vi "Arm Controller.vi"(8 "error in":errorcluster) -> ()   [LabVIEW 2017]
doc: "This VI executes continuously carrying out the current operation and responding to updates or new operations. It will often contain the timing or control code that is difficult to place directly in TeleOp. This VI generally opens all sensors and motors and isolates the rest of the robot code from knowing how the operations are carried out."
uses:
  <vilib>/Rock Robotics/WPI/Framework/Completion Status.ctl
  Arm Setpoints.ctl
  Arm Operations.ctl
  <vilib>/Rock Robotics/SystemInterfaces/DIO/FPGA_DIOPWMChannel.ctl
  <vilib>/Rock Robotics/WPI/SafetyOutput/WPI_SafetyOutputConfigMenu.ctl
  <vilib>/Rock Robotics/WPI/MotorControl/WPI_MotorControlOpen SPARK.vi
  <vilib>/Rock Robotics/Network Tables/NT Write Number.vi
panel:
  in  "Interactive Values":T1
  out "Current\nCmd":string
  in  "Buttons":cluster{"Execute Cmd":bool, "Abort Cmd":bool}
  out "Command Timing":cluster{"Start Time (ms)":u32, "Iterations":i32}
  out "Status":T3
  # "Tip: It may be helpful to observe inputs and sensor values.\nYou may also want to display tuning or debugging controls."
  # "Interactive Command: You may fill in the settings for a command\nand schedule it with the Execute button. You can observe and abort\nany command while fine tuning the code for the controller."
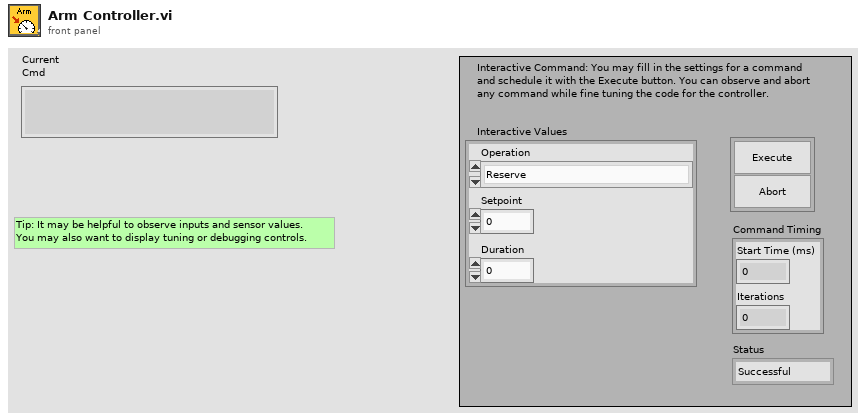
[diagram p1: front panel]
types:
  T1 = typedef "Arm Setpoints.ctl" = cluster{"Operation":T2, "Setpoint":dbl, "Duration":dbl}
  T2 = typedef "Arm Operations.ctl" = enum16{"Reserve", "Read Current", "Immediate", "Lift", "Lower"}
  T3 = typedef "Completion Status.ctl" = enum16{"Successful", "Aborted", "Incomplete"}
  T4 = typedef "WPI_SafetyOutputConfigMenu.ctl" = enum16{"Enable", "Disable"}
  T5 = typedef "FPGA_DIOPWMChannel.ctl" = enum8{"PWM 0", "PWM 1", "PWM 2", "PWM 3", "PWM 4", "PWM 5", "PWM 6", "PWM 7", "PWM 8", "PWM 9", "PWM MXP 0", "PWM MXP 1", "PWM MXP 2", "PWM MXP 3", "PWM MXP 4", "PWM MXP 5", "PWM MXP 6", "PWM MXP 7", "PWM MXP 8", "PWM MXP 9", "Invalid"}
  T6 = typedef "WPI_MotorControlDeviceRef.ctl" = cluster{"DeviceStatus":errorcluster, "Type":T7, "PWM":cluster{"PWM Channel":T5, "DeadBand":T8}, "CAN":cluster{"Device Number":u8, "SetOutput VI Ref":variant, "GetOutput VI Ref":variant, "Enable VI Ref":variant, "Disable VI Ref":variant, "Data":variant}, "Invert":bool, "DIO PWM":cluster{"PWM \"Enable\" Channel":T5, "DIOChannel":T9, "PWM Rate":dbl}}
  T7 = typedef "WPI_MotorControlType.ctl" = enum16{"PWM", "CAN", "DIO PWM"}
  T8 = typedef "WPI_PWMDeadband.ctl" = cluster{"Name":string, "maxPositivePwm":i32, "minPositivePwm":i32, "centerPwm":i32, "maxNegativePwm":i32, "minNegativePwm":i32, "angularRange":u16}
  T9 = typedef "FPGA_DIOChannel.ctl" = enum8{"DIO 0", "DIO 1", "DIO 2", "DIO 3", "DIO 4", "DIO 5", "DIO 6", "DIO 7", "DIO 8", "DIO 9", "DIO MXP 0", "DIO MXP 1", "DIO MXP 2", "DIO MXP 3", "DIO MXP 4", "DIO MXP 5", "DIO MXP 6", "DIO MXP 7", "DIO MXP 8", "DIO MXP 9", "DIO MXP 10", "DIO MXP 11", "DIO MXP 12", "DIO MXP 13", "DIO MXP 14", "DIO MXP 15", "SPI Port CS1", "SPI Port CS2", "SPI Port CS3", "SPI Port MISO", "SPI Port MOSI", "Invalid"}
  T10 = typedef "Command Status Info.ctl" = cluster{"Name":string, "Status":T3, "notifier out":T11}
  T11 = typedef "Completion Notifier.ctl" = refnum<notifier>
  T12 = cluster{"Current Command":T1, "Command Timing":cluster{"Start Time (ms)":u32, "Iterations":i32}, "Command Arguments":cluster{"Command Info":T10, "Description":string, "Default Command":T1, "queue out":refnum<queue>, "Subsystem Name":string}}
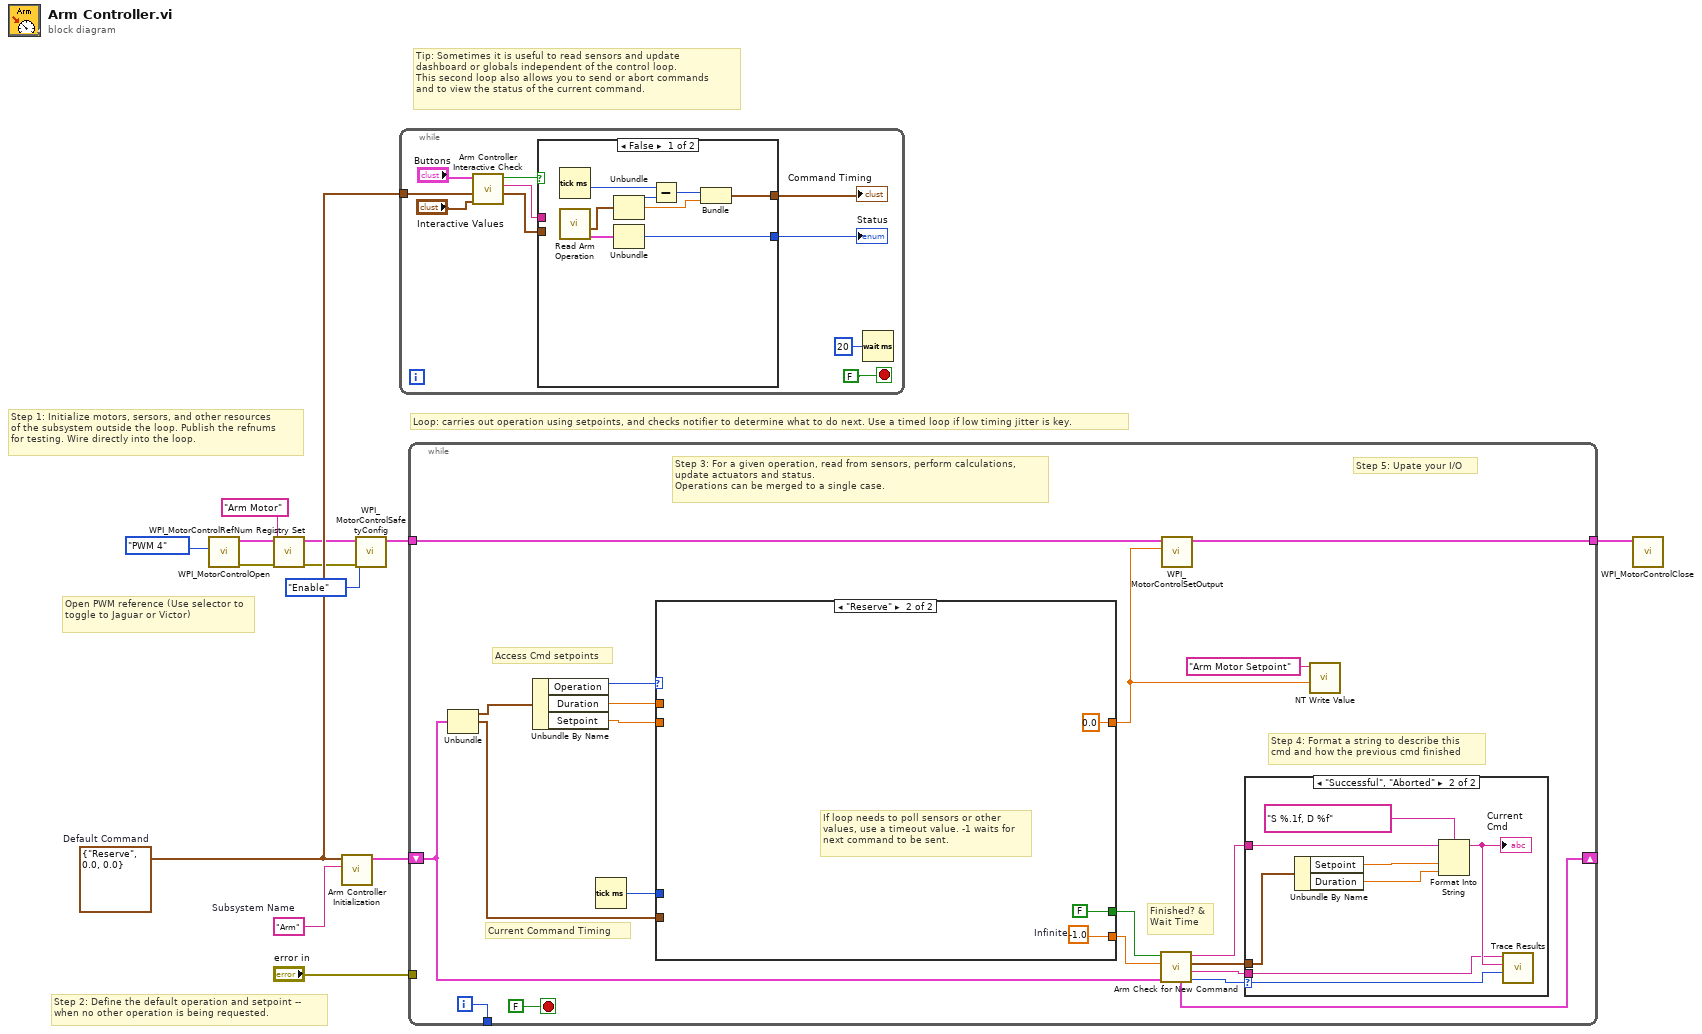
[diagram p0: block diagram]
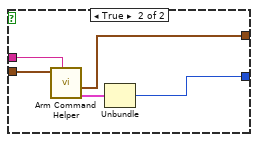
[diagram p2: hidden frame]
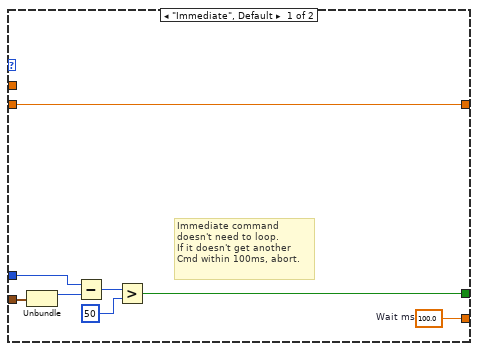
[diagram p4: hidden frame]
diagram:
  w10 = T1 {"Operation"=enum."Reserve", "Setpoint"=0.0, "Duration"=0.0}  # Default Command
  w11 = "Arm"  # Subsystem Name
  # "Open PWM reference (Use selector to toggle to Jaguar or Victor)"
  # "Tip: Sometimes it is useful to read sensors and update\ndashboard or globals independent of the control loop.\nThis second loop also allows you to send or abort commands\nand to view the status of the current command."
  # "Step 2: Define the default operation and setpoint --\nwhen no other operation is being requested."
  # "Step 1: Initialize motors, sersors, and other resources\nof the subsystem outside the loop. Publish the refnums\nfor testing. Wire directly into the loop."
  # "Loop: carries out operation using setpoints, and checks notifier to determine what to do next. Use a timed loop if low timing jitter is key."
  n1 = call-poly <vilib>:"WPI_MotorControlOpen.vi"("PWM Channel"=FPGA_DIOPWMChannel."PWM 4") -> ("error out"=w2:errorcluster, "MotorControlDeviceRef"=w8:T6)  [unwired: 3 in, 6 out]
  n2 = call <vilib>:"WPI_MotorControlRefNum Registry Set.vi"("error in (no error)"=w2, "refnum name"="Arm Motor", "MotorControlDevRef"=w8) -> ("error out"=w1:errorcluster, "MotorControlDevRef"=w7:T6)  [unwired: 7 in]
  n3 = call "Arm Controller Initialization.vi"("Subsystem Name"=w11, "Default Command"=w10) -> ("Current Command"=w12:T12)  [unwired: 9 in]
  n4 = call <vilib>:"WPI_MotorControlSafetyConfig.vi"("error in (no error)"=w1, "mode"=WPI_SafetyOutputConfigMenu."Enable", "MotorControlDevRef"=w7) -> ("MotorControlDevRef"=w6:T6)  [unwired: 7 in, 1 out]
  n5 = while {
    tunnel: w10 -> [w20]
    stop <- FALSE stop-if-true
    n6 = call "Arm Controller Interactive Check.vi"("Interactive Command in"="Interactive Values", "Default Command"=w20, "Buttons"="Buttons") -> ("Interactive Command out"=w17:T1, "Trace String"=w18:string, "Schedule"=w19:bool)  [unwired: 6 in]
    n7 = case shown="False" w19 {
      tunnel: [w31 w36] -> w16
      tunnel: w17 -> [_ w34]
      tunnel: [w27 w32] -> w15
      tunnel: w18 -> [_ w35]
      frame False {
        n8 = Tick Count (ms)() -> (millisecond timer value=w26:u32)
        n9 = call "Read Arm Operation.vi"() -> ("Command Info"=w24:T10, "SubSystem Data"=w25:T1)  [unwired: 9 in, 1 out]
        n10 = Unbundle(w25) -> ("Operation"=w30:T2, "Setpoint"=w28:dbl)  [unwired: 1 out]
        n11 = Unbundle(w24) -> ("Status"=w31:T3)  [unwired: 2 out]
        n12 = Subtract(x=w26, y=w30) -> (x-y=w29:u32)
        n13 = Bundle(w29, "Setpoint"=w28) -> (w27:cluster{u32, "Setpoint":dbl})  [unwired: 1 in]
      }
      frame True {
        n14 = call "Arm Command Helper.vi"("Description"=w35, "SubSystem Data"=w34) -> ("Command Info Out"=w33:T10, "Command Timing"=w32:cluster{"Start Time (ms)":u32, "Iterations":i32})  [unwired: 7 in, 1 out]
        n15 = Unbundle(w33) -> ("Status"=w36:T3)  [unwired: 2 out]
      }
    }
    "Status" <- w16
    "Command Timing" <- w15
    n16 = Wait (ms)(milliseconds to wait=u32 20) -> ()  [unwired: 1 out]
  }
  n17 = while {
    shift-right: [w48] -> _
    shift-left: w12 -> [w41]
    tunnel: [w55] -> _
    tunnel: "error in" -> [_]
    tunnel: w6 -> [w40]
    tunnel: [w39] -> w5
    i -> [w55]
    stop <- FALSE stop-if-true
    # "Step 5: Upate your I/O"
    # "Step 4: Format a string to describe this\ncmd and how the previous cmd finished"
    # "Current Command Timing"
    # "Access Cmd setpoints"
    # "Finished? &\nWait Time"
    # "Step 3: For a given operation, read from sensors, perform calculations,\nupdate actuators and status.\nOperations can be merged to a single case."
    n18 = Unbundle(w41) -> ("Current Command"=w54:T1, "Command Timing"=w50:cluster{"Start Time (ms)":u32, "Iterations":i32})  [unwired: 1 out]
    n19 = Unbundle By Name(w54) -> ("Operation"=w53:T2, "Duration"=w52:dbl, "Setpoint"=w49:dbl)
    n20 = Tick Count (ms)() -> (millisecond timer value=w51:u32)
    n21 = case shown="\"Reserve\"" w53 {
      tunnel: [w72 w75] -> w46
      tunnel: [w66 FALSE ("ignore previous (F)")] -> w47
      tunnel: w50 -> [w68 _]
      tunnel: w52 -> [_ _]
      tunnel: w51 -> [w67 _]
      tunnel: w49 -> [w65 _]
      tunnel: [w65 0.0 ("Setpoint")] -> w38
      frame "Immediate", Default {
        w72 = 100.0  # Wait ms
        # "Immediate command\ndoesn't need to loop.\nIf it doesn't get another\nCmd within 100ms, abort."
        n22 = Unbundle(w68) -> ("Start Time (ms)"=w71:u32)  [unwired: 1 out]
        n23 = Subtract(x=w67, y=w71) -> (x-y=w70:u32)
        n24 = Greater?(x=w70, y=u8 50 ("Left Motor")) -> (0:w66:bool)
      }
      frame "Reserve" {
        w75 = -1.0  # Infinite
        # "If loop needs to poll sensors or other\nvalues, use a timeout value. -1 waits for\nnext command to be sent."
      }
    }
    n25 = call "Arm Check for New Command.vi"("Current Command"=w41, "Wait time (ms)"=w46, "Finished?"=w47) -> ("Completion"=w42:T3, "Subsystem Name"=w43:string, "Current Command"=w44:T1, "Initial Trace String"=w45:string, "NextCommand"=w48:T12)  [unwired: 4 in]
    n26 = call <vilib>:"WPI_MotorControlSetOutput.vi"("Output"=w38, "MotorControlDevRef"=w40) -> ("MotorControlDevRef"=w39:T6)  [unwired: 2 in, 7 out]
    n27 = case shown="\"Successful\", \"Aborted\"" w42 {
      selector: w42 -> [_ w64]
      tunnel: w45 -> [_ w60]
      tunnel: w44 -> [_ w61]
      tunnel: w43 -> [_ w57]
      frame "Incomplete", Default {
        # "Continuing current command"
      }
      frame "Successful", "Aborted" {
        # "Report and setup for next command"
        n28 = Unbundle By Name(w61) -> ("Setpoint"=w63:dbl, "Duration"=w58:dbl)
        n29 = Format Into String(format string="S %.1f, D %f", initial string=w60, w63, w58) -> (resulting string=w59:string)  [unwired: 1 in, 1 out]
        "Current\nCmd" <- w59
        n30 = call <vilib>:"Trace Results.vi"("Status of previous command"=w64, "Description"=w59, "Subsystem"=w57) -> ()  [unwired: 9 in]
      }
    }
    n31 = call-poly <vilib>:"NT Write Value.vi"("Numeric"=w38, "Name"="Arm Motor Setpoint") -> ()  [unwired: 9 in, 1 out]
  }
  n32 = call <vilib>:"WPI_MotorControlClose.vi"("MotorControlDevRef"=w5) -> ()  [unwired: 1 in, 10 out]
